vi "Read connection ID.vi"(8 "error in (no error)":errorcluster, 11 "KinesisCube in":refnum<class "KinesisCube.lvclass">) -> (0 "error out":errorcluster, 2 "connection ID":refnum<k24>, 3 "KinesisCube out":refnum<class "KinesisCube.lvclass">)   [LabVIEW 2020, in "KinesisCube.lvclass"]
uses:
  KinesisCube.lvclass
  C:/GEECS/Developers Version/builds/Device builds/KinesisCube/Thorlabs.MotionControl.KCube.PiezoCLI.dll
  Thorlabs.MotionControl.KCube.PiezoCLI.dll
  KinesisCube.lvclass/KinesisCube.ctl
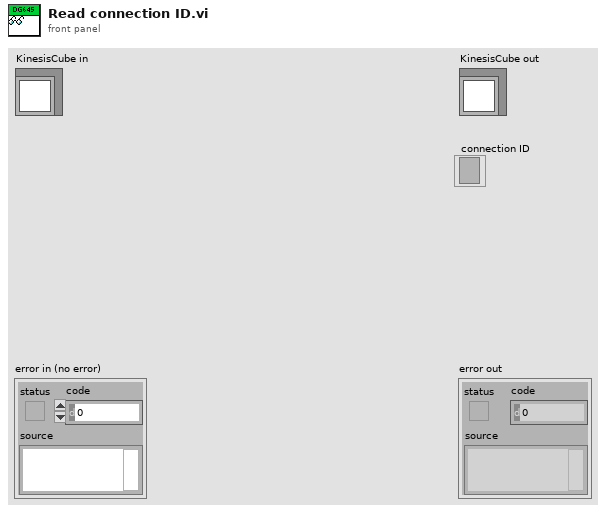
[diagram p1: front panel]
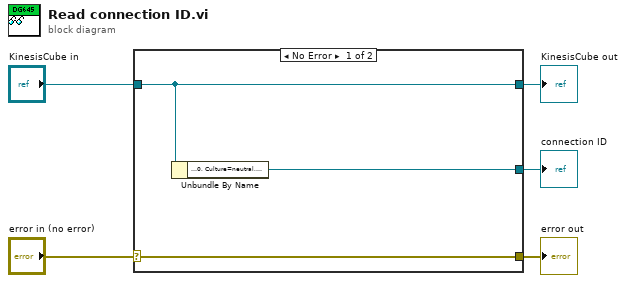
[diagram p0: block diagram]
diagram:
  n1 = case shown="No Error" "error in (no error)" {
    selector: "error in (no error)" -> [w8 w9]
    tunnel: [w8 w9] -> w4
    tunnel: [w7 w10] -> w2
    tunnel: "KinesisCube in" -> [w7 w10]
    tunnel: [w6 _] -> w1
    frame No Error {
      n2 = Unbundle By Name(w7) -> ("connection ID"=w6:refnum<k24>)
    }
    frame Error {
    }
  }
  "error out" <- w4
  "KinesisCube out" <- w2
  "connection ID" <- w1
